vi "ThresholdSweepL0.vi"() -> ()   [LabVIEW 2012]
uses:
  <vilib>/Utility/NIReport.llb/NI_report.lvclass
  <vilib>/Utility/NIReport.llb/HTML/NI_HTML.lvclass
  <instrlib>/Agilent 8000 Series/Public/Configure/Configure Math (Binary Operation).vi
  L0&L1/L0_BOARD_TESTs/trunk/Sum_Abrilader/L0_Sum_Adder Folder/C/Program Files/National Instruments/LabVIEW 2012/instr.lib/Agilent 8000 Series/Public/Data/Low Level/Fetch Measurement (More).vi
  <instrlib>/Agilent 8000 Series/Agilent 8000 Series.lvlib
panel:
  in  "Serial Number":string="SN_029_L0"
  out "Current Channel":i32=6
  in  "Step":i32=1
  out "Current Threshold":i32=190
  in  "Upper Thresold":i32=200
  in  "Lower Threshold":i32=400
  in  "Channels":i32[](array[numeric])=[0, 1, 2, 3, 4, 5, 6]
  in  "IPR?":bool=TRUE
  out "Data":string="empty_read_buffer0_2-65@1\r\n0_2-76@0\r\n"
  out "IPR_count":u32
  in  "Sum/Maj 2":bool
  in  "Gen Active":bool=TRUE
  in  "Control\nGenNOsc":bool=TRUE
  in  "Amp Scaler":dbl(slide)=15.152261545188344 scale=0.1..125.0
  in  "Voltage Input":dbl=0.3
  in  "Sum/Maj":bool
  in  "Ib Clip select":i32(slide)=63 scale=0.0..63.0
  in  "Clipping Select":i32(slide)=1 scale=1.0..3.0
  in  "Attenuation Select":i32(slide) scale=0.0..15.0
  in  "Delay Enable":i32(slide) scale=0.0..31.0
  in  "Instrument VISA in":T1={"AWG VISA"="AgilentGenerator1", "Oscilloscope  VISA "="AgilentOsciloscope", "Integration Board IP"="172.16.17.47", "connection ID"=refnum, "report out"=refnum, "report file path"=path "C:/Users/omartinez/Desktop/L0nL1_Results"}
  out "error out":errorcluster
  in  "error in":errorcluster
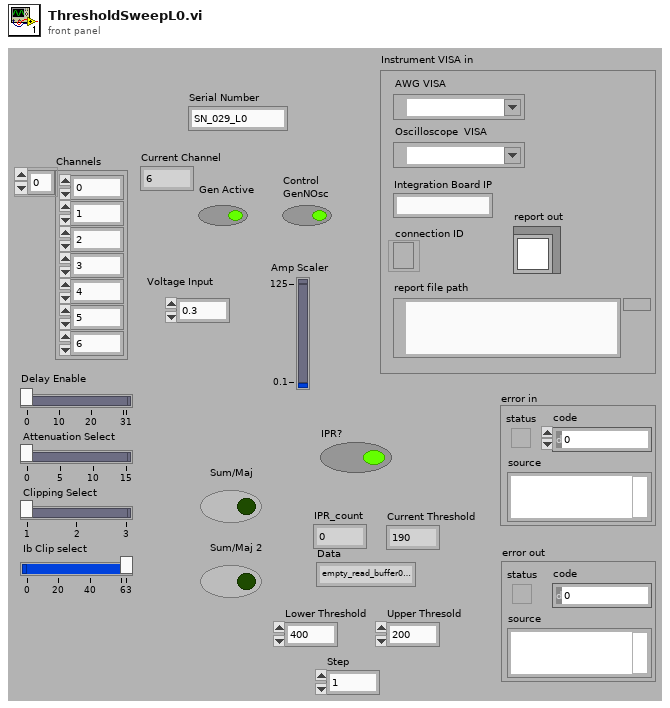
[diagram p1: front panel]
types:
  T1 = cluster{"AWG VISA":refnum<visa-resource-name>, "Oscilloscope  VISA ":refnum<visa-resource-name>, "Integration Board IP":string, "connection ID":refnum<k5>, "report out":refnum<class "NI_report.lvclass">, "report file path":path}
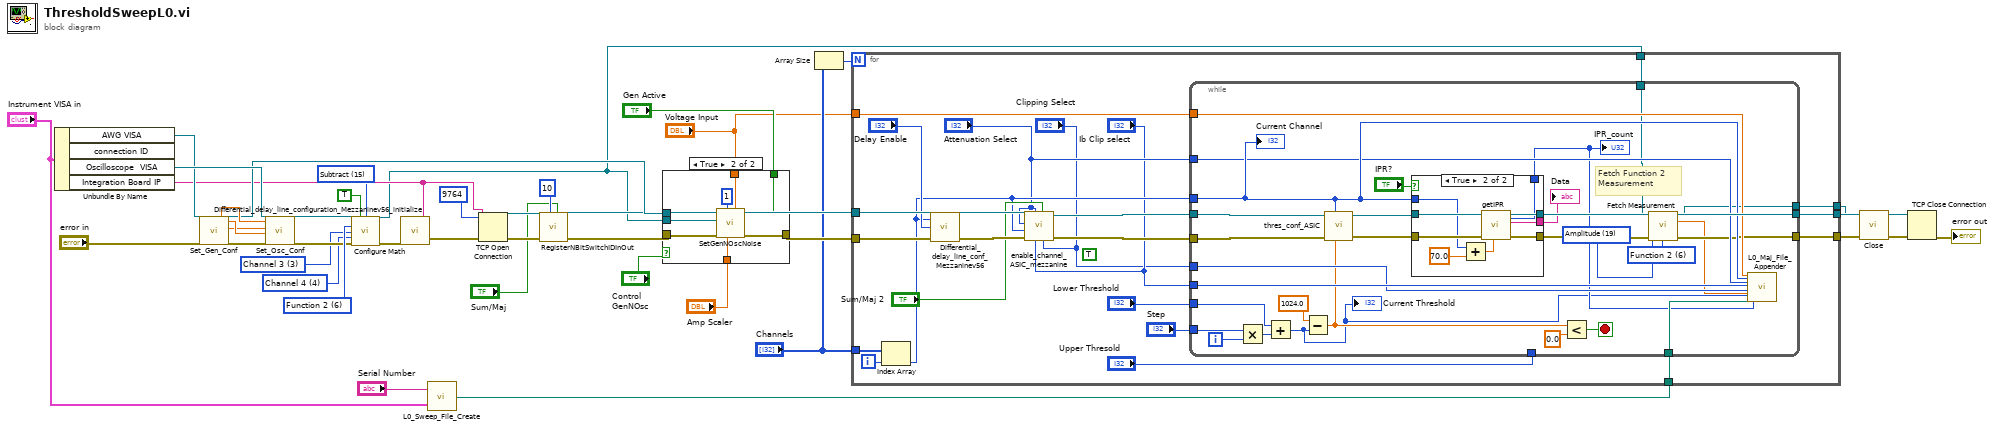
[diagram p0: block diagram]
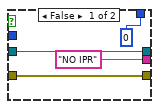
[diagram p2: hidden frame]
diagram:
  w27 = u16 6 items=["Function 1"=5, "Function 2"=6, "Function 3"=7, "Function 4"=8] ("Math Channel (5: Function 1)")
  w28 = u16 15 items=["Add"=12, "Divide"=13, "Multiply"=14, "Subtract"=15, "Common Mode"=16, "Versus"=17] ("Math Operation (12: Add)")
  w22 = 3 items=["Channel 1"=1, "Channel 2"=2, "Channel 3"=3, "Channel 4"=4] ("Channel (1: Channel 1)")
  w23 = 4 items=["Channel 1"=1, "Channel 2"=2, "Channel 3"=3, "Channel 4"=4] ("Channel (1: Channel 1)")
  n1 = Unbundle By Name("Instrument VISA in") -> ("AWG VISA"=w37:refnum<visa-resource-name>, "Oscilloscope  VISA"=w38:refnum<visa-resource-name>, "Integration Board IP"=w30:string)  [unwired: 1 out]
  n2 = call "Set_Gen_Conf.vi"("AWG VISA"=w37, "error in (no error)"="error in") -> ("Amplitude 1 OUT"=w35:dbl, "VISA resource name out"=w31:refnum<visa-resource-name>, "Pulse Width in seconds 1 OUT"=w34:dbl, "Trigger Level 1"=w33:dbl, "error out"=w39:errorcluster)  [unwired: 10 in, 3 out]
  n3 = call "Set_Osc_Conf.vi"("VISA resource name"=w38, "Amplitude IN"=w35, "Trigger Level IN"=w33, "Pulse Width in seconds IN"=w34, "error in (no error)"=w39) -> ("VISA resource name out"=w26:refnum<visa-resource-name>, "error out"=w25:errorcluster)  [unwired: 13 in]
  n4 = call-poly <instrlib>:"Configure Math.vi"("VISA resource name"=w26, "Enable Math Channel (T:Enable)"=TRUE, "Math Operation (12: Add)"=w28, "Math Channel (5: Function 1)"=w27, "Math Operand (1: Channel 1)"=w22, "Math Operand (2: Channel 2)"=w23, "error in (no error)"=w25) -> ("VISA resource name out"=w4:refnum<visa-resource-name>, "error out"=w24:errorcluster)  [unwired: 7 in]
  n5 = call "Differential_delay_line_configuration_Mezzaninev56_initialize.vi"("error in (no error)"=w24, "address"=w30) -> ("error out 2"=w32:errorcluster)
  n6 = call "L0_Sweep_File_Create.vi"("input cluster"="Instrument VISA in", "Serial Number"="Serial Number") -> ("appended path"=w6:path)
  n7 = TCP Open Connection(address=w30, remote port or service name=9764, error in (no error)=w32) -> (connection ID=w18:refnum<k5>, error out=w20:errorcluster)  [unwired: 2 in]
  n8 = call "RegisterNBitSwitchIDInOut.vi"("Switch Bit"="Sum/Maj", "N Bit"=10, "error in (no error)"=w20, "connection ID"=w18) -> ("error out"=w19:errorcluster, "connection ID out"=w17:refnum<k5>)  [unwired: 5 in]
  n9 = case shown="True" "Control\nGenNOsc" {
    tunnel: w4 -> [_ w50]
    tunnel: w31 -> [_ w49]
    tunnel: w19 -> [w42 w48]
    tunnel: [w42 w47] -> w14
    tunnel: "Voltage Input" -> [_ w45]
    tunnel: "Amp Scaler" -> [_ w44]
    tunnel: "Gen Active" -> [_ w43]
    frame False {
    }
    frame True {
      n10 = call "SetGenNOscNoise.vi"("Enable Output"=w43, "Input Voltage"=w45, "Amp Scaler"=w44, "NChannels"=1, "error in (no error)"=w48, "VISA resource name"=w50, "AWG VISA"=w49) -> ("error out 2"=w47:errorcluster)  [unwired: 4 in]
    }
  }
  n11 = Array Size(array="Channels") -> (size(s)=w10:i32)
  n12 = for {
    N: w10 -> [_]
    tunnel: [w73] -> w2
    tunnel: w17 -> [w72]
    tunnel: [w71] -> w15
    tunnel: w14 -> [w70]
    tunnel: "Channels" -> [w65]
    tunnel: w6 -> [w57]
    tunnel: "Voltage Input" -> [w56]
    tunnel: w4 -> [w52]
    tunnel: [w51] -> w1
    i -> [w64]
    (unwired) TRUE ("CompBuf_en_b")
    n13 = Index Array(array=w65, index=w64) -> (element=w63:i32)
    n14 = call "Differential_delay_line_conf_Mezzaninev56.vi"("connection ID"=w72, "channel"=w63, "Delay value"="Delay Enable", "error in (no error)"=w70) -> ("connection ID out"=w68:refnum<k5>, "error out 2"=w69:errorcluster)  [unwired: 4 in, 6 out]
    n15 = call "enable_channel_ASIC_mezzanine.vi"("Clip_sel_b"="Clipping Select", "maj/sum"="Sum/Maj 2", "Ib_clipVb"="Ib Clip select", "Att gain"="Attenuation Select", "error in"=w69, "Channel"=w63, "id_in"="Attenuation Select", "connection ID"=w68) -> ("error out"=w59:errorcluster, "connection ID out"=w58:refnum<k5>)  [unwired: 1 in, 1 out]
    n16 = while {
      tunnel: [w81] -> w73
      tunnel: [w103] -> w71
      tunnel: w59 -> [w102]
      tunnel: w58 -> [w101]
      tunnel: w63 -> [w89]
      tunnel: "Lower Threshold" -> [w97]
      tunnel: "Upper Thresold" -> [_]
      tunnel: "Step" -> [w93]
      tunnel: w57 -> [w91]
      tunnel: w56 -> [w90]
      tunnel: "Attenuation Select" -> [w88]
      tunnel: "Ib Clip select" -> [w87]
      tunnel: "Clipping Select" -> [w86]
      tunnel: w52 -> [w80]
      tunnel: [w79] -> w51
      i -> [w94]
      stop <- w96 stop-if-true
      w84 = 19 items=["Rise Time", "Fall Time", "Frequency", "Period", "Voltage RMS(AC)", "Voltage RMS(DC)", "Voltage RMS (AC,cycle)", "Voltage RMS (DC,cycle)", "Voltage Max", "Voltage Min", "Voltage Middle", "Voltage Vpp", "Voltage High", "Voltage Low", "Voltage Average", "Voltage Average (cycle)", "Width Negative", "Width Positive", "Duty Cycle Positive", "Amplitude", "Overshoot", "Preshoot", "Voltage Base", "Voltage Upper", "Time Max", "Time Min", "Color Grade Crossing", "Color Grade Eye Width", "Color Grade Eye Height", "Color Grade Eye Q-Factory", "Color Grade Eye Duty Cycle Distortion(Percent)", "Color Grade Eye Duty Cycle Distortion(Time)", "Color Grade Eye Jitter(PP)", "Color Grade Eye Width(RMS)", "Cycle-cycle Duty Jitter(Rising)", "Cycle-cycle Duty Jitter(Falling)", "Cycle-cycle Jitter(Rising)", "Cycle-cycle Jitter(Falling)", "Cycle-cycle - Width", "Cycle-cycle + Width", "Date Rate", "Unit Interval", "FFT Delta Frequency", "FFT Delta Magnitude", "FFT Frequency", "FFT Magnitude", "Slew Rate", "Area (Entire Display)", "Area(Single Cycle)", "Duty Cycle (Rising)", "Duty Cycle (Falling)"] ("Measurement Function (0: Rise Time)")
      w83 = 6 items=["Channel 1"=1, "Channel 2"=2, "Channel 3"=3, "Channel 4"=4, "Function 1"=5, "Function 2"=6, "Function 3"=7, "Function 4"=8, "Memory 1"=9, "Memory 2"=10, "Memory 3"=11, "Memory 4"=12] ("Channel (1: Channel 1)")
      # "Fetch Function 2\nMeasurement"
      n17 = Multiply(x=w93, y=w94) -> (x*y=w95:i32)
      n18 = Add(x=w97, y=w95) -> (x+y=w74:i32)
      "Current Threshold" <- w74
      n19 = Subtract(x=1024.0, y=w74) -> (x-y=w77:dbl)
      n20 = call "thres_conf_ASIC.vi"("threshold"=w77, "Ring"=w89, "error out 3"=w102, "connection ID"=w101) -> ("error out 2"=w92:errorcluster, "connection ID out"=w98:refnum<k5>)  [unwired: 4 in, 2 out]
      n21 = case shown="True" "IPR?" {
        tunnel: w92 -> [w107 w116]
        tunnel: [w107 w108] -> w82
        tunnel: w98 -> [w106 w115]
        tunnel: [w106 w114] -> w103
        tunnel: [u32 0 ("IPR_count") w111] -> w85
        tunnel: ["NO IPR" ("Data") w110] -> w100
        tunnel: w89 -> [_ w109]
        frame False {
        }
        frame True {
          n22 = Add(x=w109, y=70.0) -> (x+y=w113:dbl)
          n23 = call "getIPR.vi"("Address"=w113, "error in"=w116, "connection ID"=w115) -> ("error out"=w108:errorcluster, "Data"=w110:string, "connection ID out"=w114:refnum<k5>, "IPR_count"=w111:u32)  [unwired: 5 in]
        }
      }
      "IPR_count" <- w85
      "Data" <- w100
      n24 = Less?(x=w77, y=0.0) -> (x < y?=w96:bool)
      n25 = call-poly "Fetch Measurement.vi"("VISA resource name"=w80, "Channel (1: Channel 1)"=w83, "Measurement Function (0: Rise Time)"=w84, "error in (no error)"=w82) -> ("VISA resource name out"=w79:refnum<visa-resource-name>, "Measurement"=w78:dbl, "error out"=w81:errorcluster)  [unwired: 9 in]
      n26 = call "L0_Maj_File_Appender.vi"("Vin"=w90, "CH"=w89, "Att"=w88, "IbClip"=w87, "Clip"=w86, "Vmeas"=w78, "Threshold"=w74, "file path (dialog if empty)"=w91, "DT"=w85) -> ()  [unwired: 19 in]
      "Current Channel" <- w89
    }
  }
  n27 = call <instrlib>:"Close.vi"("error in (no error)"=w2, "VISA resource name"=w1) -> ("error out"=w3:errorcluster)  [unwired: 9 in]
  n28 = TCP Close Connection(connection ID=w15, error in (no error)=w3) -> (error out=→"error out":errorcluster)  [unwired: 1 in, 1 out]
